vi "CreateControlRecord.vi"(6 "Pass_Through_Time":dbl=-1.0 format="%-33.4f", 10 "Control Record Payload Data":T2, 11 "ControlRecordType":T1) -> (3 "control record":u8[](array[numeric]) format="%x")   [LabVIEW 2023]
uses:
  impl_ControlRecordType_ENUM.ctl
  <vilib>/Rock Robotics/WPI/ThirdParty/JAS_Junk/TrajLib/VI/Util_GetTime_U32.vi
  <vilib>/Rock Robotics/WPI/ThirdParty/JAS_Junk/TrajLib/VI/Util_GetTime_U64.vi
  <vilib>/Rock Robotics/WPI/ThirdParty/JAS_Junk/TrajLib/Trajectory_Library.lvlib
panel:
  out "payload data (little endian)":u8[](array[numeric]) format="%x"
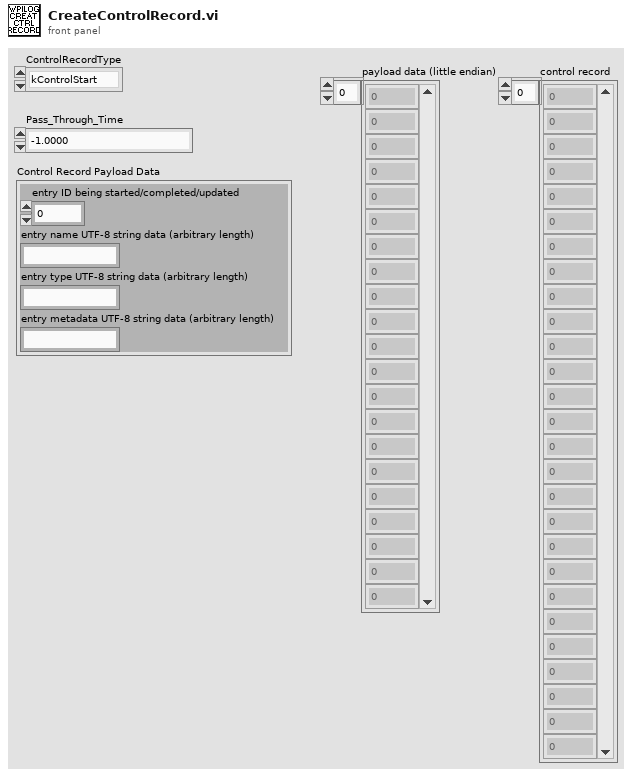
[diagram p1: front panel]
types:
  T1 = typedef "impl_ControlRecordType_ENUM.ctl" = enum16{"kControlStart", "kControlFinish", "kControlSetMetadata"}
  T2 = cluster{"entry ID being started/completed/updated":i32, "entry name UTF-8 string data (arbitrary length)":string, "entry type UTF-8 string data (arbitrary length)":string, "entry metadata UTF-8 string data (arbitrary length)":string}
  T3 = enum16{"big-endian, network order", "native, host order", "little-endian"}
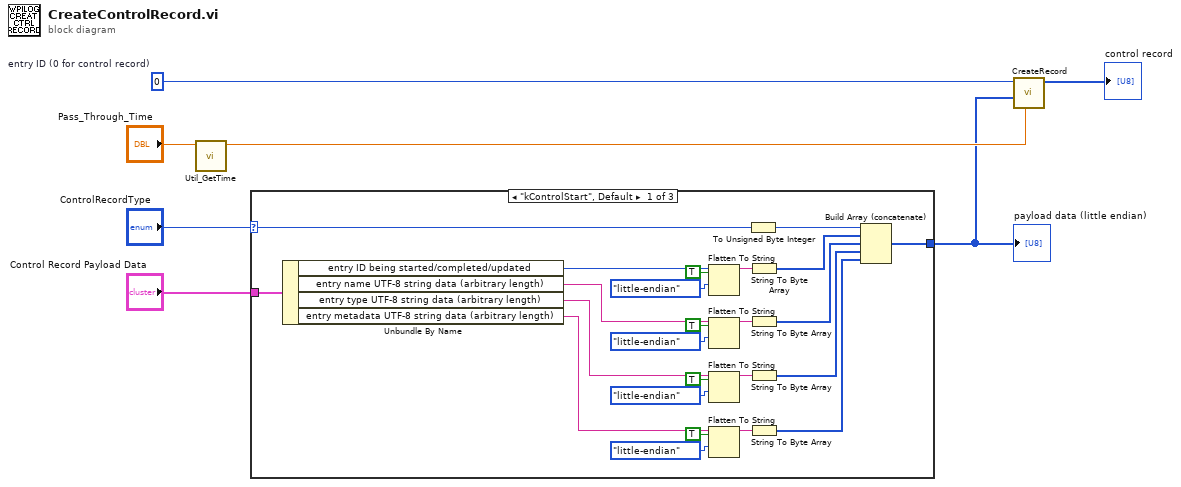
[diagram p0: block diagram]
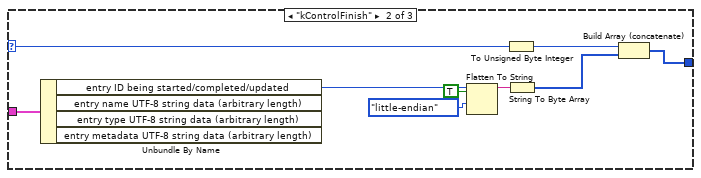
[diagram p2: hidden frame]
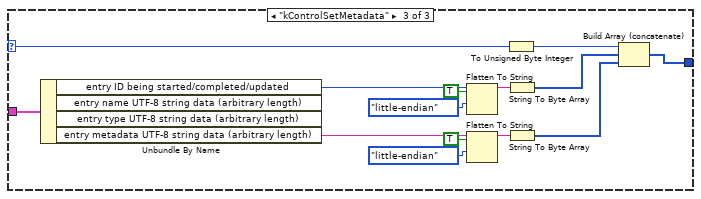
[diagram p3: hidden frame]
diagram:
  w6 = 0  # entry ID (0 for control record)
  n1 = call <vilib>:"Util_GetTime.vi"("Pass_Through_Time"="Pass_Through_Time") -> ("FPGA_Time_Seconds"=w4:dbl)  [unwired: 8 in, 2 out]
  n2 = case shown="\"kControlStart\", Default" "ControlRecordType" {
    selector: "ControlRecordType" -> [w31 w40 w54]
    tunnel: "Control Record Payload Data" -> [w29 w38 w52]
    tunnel: [w8 w32 w41] -> w2
    frame "kControlStart", Default {
      n3 = Unbundle By Name(w29) -> ("entry ID being started/completed/updated"=w10:i32, "entry name UTF-8 string data (arbitrary length)"=w19:string, "entry type UTF-8 string data (arbitrary length)"=w17:string, "entry metadata UTF-8 string data (arbitrary length)"=w16:string)
      n4 = Flatten To String(anything=w10, prepend array or string size? (T)=TRUE, byte order (0:big-endian, network order)=T3."little-endian") -> (data string=w11:string)  [unwired: 1 in, 2 out]
      n5 = Flatten To String(anything=w19, prepend array or string size? (T)=TRUE, byte order (0:big-endian, network order)=T3."little-endian") -> (data string=w28:string)  [unwired: 1 in, 2 out]
      n6 = Flatten To String(anything=w17, prepend array or string size? (T)=TRUE, byte order (0:big-endian, network order)=T3."little-endian") -> (data string=w25:string)  [unwired: 1 in, 2 out]
      n7 = Flatten To String(anything=w16, prepend array or string size? (T)=TRUE, byte order (0:big-endian, network order)=T3."little-endian") -> (data string=w21:string)  [unwired: 1 in, 2 out]
      n8 = To Unsigned Byte Integer(number=w31) -> (unsigned 8bit integer=w30:u8)
      n9 = String To Byte Array(string=w11) -> (unsigned byte array=w9:u8[])
      n10 = String To Byte Array(string=w28) -> (unsigned byte array=w18:u8[])
      n11 = String To Byte Array(string=w25) -> (unsigned byte array=w15:u8[])
      n12 = String To Byte Array(string=w21) -> (unsigned byte array=w14:u8[])
      n13 = Build Array (concatenate)(w30, w9, w18, w15, w14) -> (w8:u8[])
    }
    frame "kControlFinish" {
      n14 = Unbundle By Name(w38) -> ("entry ID being started/completed/updated"=w34:i32)  [unwired: 3 out]
      n15 = Flatten To String(anything=w34, prepend array or string size? (T)=TRUE, byte order (0:big-endian, network order)=T3."little-endian") -> (data string=w35:string)  [unwired: 1 in, 2 out]
      n16 = To Unsigned Byte Integer(number=w40) -> (unsigned 8bit integer=w39:u8)
      n17 = String To Byte Array(string=w35) -> (unsigned byte array=w33:u8[])
      n18 = Build Array (concatenate)(w39, w33) -> (w32:u8[])
    }
    frame "kControlSetMetadata" {
      n19 = Unbundle By Name(w52) -> ("entry ID being started/completed/updated"=w44:i32, "entry metadata UTF-8 string data (arbitrary length)"=w48:string)  [unwired: 2 out]
      n20 = Flatten To String(anything=w44, prepend array or string size? (T)=TRUE, byte order (0:big-endian, network order)=T3."little-endian") -> (data string=w45:string)  [unwired: 1 in, 2 out]
      n21 = Flatten To String(anything=w48, prepend array or string size? (T)=TRUE, byte order (0:big-endian, network order)=T3."little-endian") -> (data string=w50:string)  [unwired: 1 in, 2 out]
      n22 = To Unsigned Byte Integer(number=w54) -> (unsigned 8bit integer=w53:u8)
      n23 = String To Byte Array(string=w45) -> (unsigned byte array=w43:u8[])
      n24 = String To Byte Array(string=w50) -> (unsigned byte array=w42:u8[])
      n25 = Build Array (concatenate)(w53, w43, w42) -> (w41:u8[])
    }
  }
  "payload data (little endian)" <- w2
  n26 = call "CreateRecord.vi"("Pass_Through_Time"=w4, "payload data (little endian)"=w2, "entry ID"=w6) -> ("record"=→"control record":u8[])  [unwired: 8 in]
